vi "Read Measurement (More).vi"(0 "VISA resource name":refnum<visa-resource-name>, 5 "Measurement Source (1: Channel 1)":i32(ring)=1 caption="Channel (1: Channel 1)" items=["Channel 1"=1, "Channel 2"=2, "Channel 3"=3, "Channel 4"=4, "Function 1"=5, "Function 2"=6, "Function 3"=7, "Function 4"=8, "Memory 1"=9, "Memory 2"=10, "Memory 3"=11, "Memory 4"=12, "Clock"=15, "MTrend"=16, "MSpectrum"=17, "Equalized"=18, "DIG 0"=20, "DIG 1"=21, "DIG 2"=22, "DIG 3"=23, "DIG 4"=24, "DIG 5"=25, "DIG 6"=26, "DIG 7"=27, "DIG 8"=28, "DIG 9"=29, "DIG 10"=30, "DIG 11"=31, "DIG 12"=32, "DIG 13"=33, "DIG 14"=34, "DIG 15"=35], 7 "Measurement Function (0: Rise Time)":i32(ring) items=["Rise Time", "Fall Time", "Frequency", "Period", "Voltage RMS (AC)", "Voltage RMS (DC)", "Voltage RMS (AC,cycle)", "Voltage RMS (DC,cycle)", "Voltage Max", "Voltage Min", "Voltage Middle", "Voltage Vpp", "Voltage High", "Voltage Low", "Voltage Average", "Voltage Average (cycle)", "Width Negative", "Width Positive", "Duty Cycle Positive", "Amplitude", "Overshoot", "Preshoot", "Voltage Base", "Voltage Upper", "Time Max", "Time Min", "Color Grade Crossing", "Color Grade Eye Width", "Color Grade Eye Height", "Color Grade Eye Q-Factory", "Color Grade Eye Duty Cycle Distortion (Percent)", "Color Grade Eye Duty Cycle Distortion (Time)", "Color Grade Eye Jitter (PP)", "Color Grade Eye Width (RMS)", "Cycle-cycle Duty Jitter (Rising)", "Cycle-cycle Duty Jitter (Falling)", "Cycle-cycle Jitter (Rising)", "Cycle-cycle Jitter (Falling)", "Cycle-cycle - Width", "Cycle-cycle + Width", "Date Rate", "Unit Interval", "FFT Delta Frequency", "FFT Delta Magnitude", "FFT Frequency", "FFT Magnitude", "Slew Rate", "Area (Entire Display)", "Area (Single Cycle)", "Duty Cycle (Rising)", "Duty Cycle (Falling)", "Clock Recovery Rate", "Color Grade Eye Height (Measured)", "Color Grade Eye Height (Extrapolated)", "Color Grade Eye Width (Measured)", "Color Grade Eye width (Extrapolated)"], 9 "Maximum Time (10000ms)":u32=10000, 11 "error in (no error)":errorcluster) -> (4 "VISA resource name out":refnum<visa-resource-name>, 6 "Measurement":dbl, 15 "error out":errorcluster)   [LabVIEW 2020, in "Agilent 90000 Series.lvlib"]
doc: "Initiates an acquisition on the channels that you enable with the Configure Channel VI. It then waits for the acquisition to complete, obtains a waveform measurement on the channel you specify, and returns the measurement value. You specify a particular measurement type, such as rise time, frequency, and voltage peak-to-peak. You can call the Fetch Waveform Measurement VI separately for any other waveform measurement that you want to obtain on a specific channel without initiating another acquisition."
uses:
  Agilent 90000 Series.lvlib
  Low Level/Fetch Measurement (More).vi
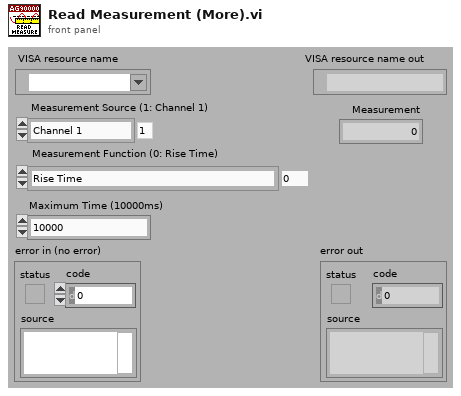
[diagram p1: front panel]
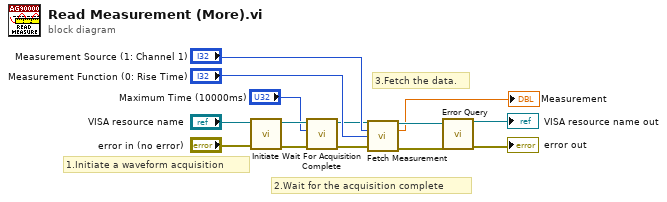
[diagram p0: block diagram]
diagram:
  # "3.Fetch the data."
  # "2.Wait for the acquisition complete"
  # "1.Initiate a waveform acquisition"
  n1 = call "Initiate.vi"("error in (no error)"="error in (no error)", "VISA resource name"="VISA resource name") -> ("error out"=w6:errorcluster, "VISA resource name out"=w7:refnum<visa-resource-name>)  [unwired: 8 out]
  n2 = call "Wait For Acquisition Complete.vi"("error in (no error)"=w6, "Maximum Time (10000ms)"="Maximum Time (10000ms)", "VISA resource name"=w7) -> ("error out"=w1:errorcluster, "VISA resource name out"=w2:refnum<visa-resource-name>)  [unwired: 7 out]
  n3 = call-poly "Fetch Measurement.vi"("VISA resource name"=w2, "Measurement Source (1: Channel 1)"="Measurement Source (1: Channel 1)", "Measurement Function (0: Rise Time)"="Measurement Function (0: Rise Time)", "error in (no error)"=w1) -> ("VISA resource name out"=w10:refnum<visa-resource-name>, "Measurement"=→"Measurement":dbl, "error out"=w9:errorcluster)  [unwired: 1 in, 8 out]
  n4 = call "Error Query.vi"("error in (no error)"=w9, "VISA resource name"=w10) -> ("error out"=→"error out":errorcluster, "VISA resource name out"=→"VISA resource name out":refnum<visa-resource-name>)  [unwired: 8 out]
